vi "Jog Z_o.vi"(10 "array IN":dbl[](array[numeric]), 11 "Jog Cluster":T1={"Jog XY Cluster"={"object goes up"=FALSE, "object goes down"=FALSE, "object goes right"=FALSE, "object goes left"=FALSE, "SW2"=FALSE, "SW1"=FALSE, "YY (mm)"=0.1, "YN (mm) "=0.01, "NY (mm) "=0.005, "NN (mm) "=0.001}, "Jog Z Cluster "={"Z go down 0.1 mm"=FALSE, "Z go up 0.1 mm"=FALSE, "Z go down 0.05 mm"=FALSE, "Z go up 0.05 mm"=FALSE, "Z go down 0.01 mm"=FALSE, "Z go up 0.01 mm"=FALSE, "Z go down"=FALSE, "Z go up"=FALSE, "step (mm)"=0.001}}) -> (2 "array OUT":dbl[](array[numeric]), 3 "Jog Cluster 2":T1={"Jog XY Cluster"={"object goes up"=FALSE, "object goes down"=FALSE, "object goes right"=FALSE, "object goes left"=FALSE, "SW2"=FALSE, "SW1"=FALSE, "YY (mm)"=0.1, "YN (mm) "=0.01, "NY (mm) "=0.005, "NN (mm) "=0.001}, "Jog Z Cluster "={"Z go down 0.1 mm"=FALSE, "Z go up 0.1 mm"=FALSE, "Z go down 0.05 mm"=FALSE, "Z go up 0.05 mm"=FALSE, "Z go down 0.01 mm"=FALSE, "Z go up 0.01 mm"=FALSE, "Z go down"=FALSE, "Z go up"=FALSE, "step (mm)"=0.001}})   [LabVIEW 2016]
panel:
  out "output array":dbl[](array[numeric])
  out "element":dbl
  out "index of element":i32
  out "appended array":bool[](array[boolean])
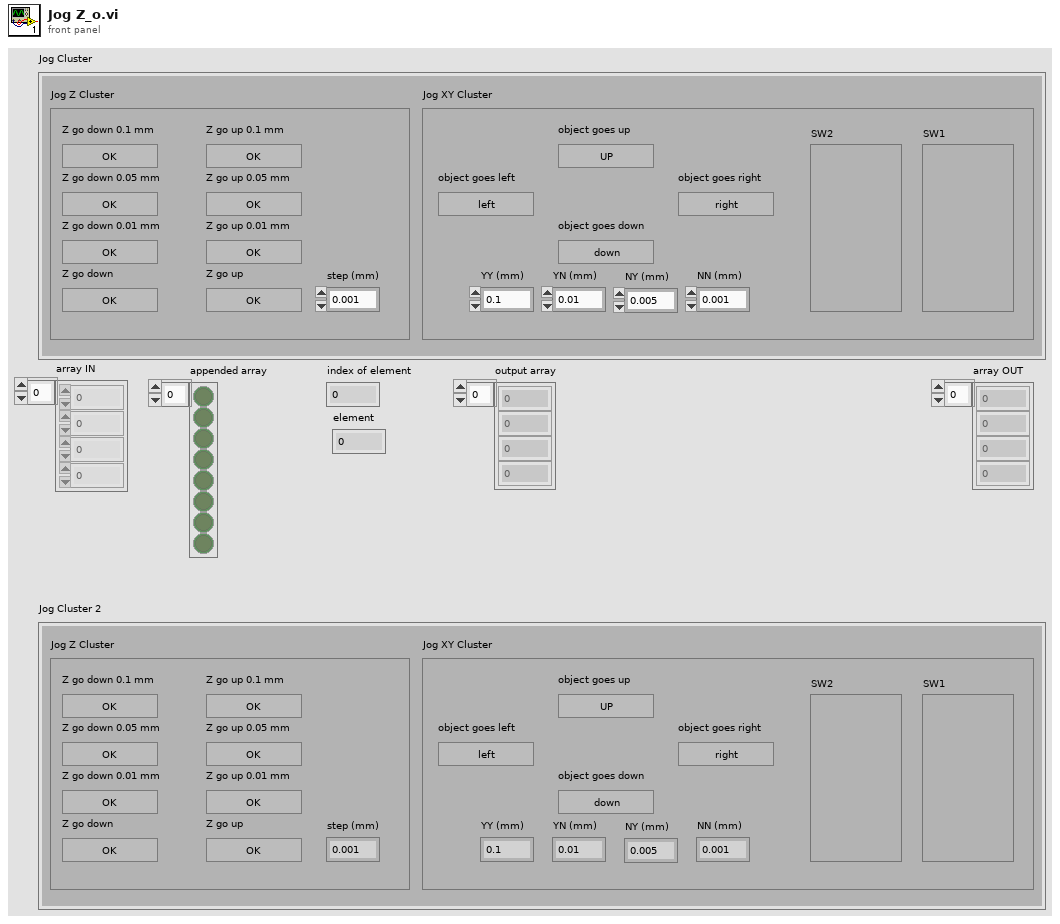
[diagram p1: front panel]
types:
  T1 = cluster{"Jog XY Cluster":cluster{"object goes up":bool, "object goes down":bool, "object goes right":bool, "object goes left":bool, "SW2":bool, "SW1":bool, "YY (mm)":dbl, "YN (mm) ":dbl, "NY (mm) ":dbl, "NN (mm) ":dbl}, "Jog Z Cluster ":cluster{"Z go down 0.1 mm":bool, "Z go up 0.1 mm":bool, "Z go down 0.05 mm":bool, "Z go up 0.05 mm":bool, "Z go down 0.01 mm":bool, "Z go up 0.01 mm":bool, "Z go down":bool, "Z go up":bool, "step (mm)":dbl}}
  T2 = cluster{"Z go down 0.1 mm":bool, "Z go up 0.1 mm":bool, "Z go down 0.05 mm":bool, "Z go up 0.05 mm":bool, "Z go down 0.01 mm":bool, "Z go up 0.01 mm":bool, "Z go down":bool, "Z go up":bool, "step (mm)":dbl}
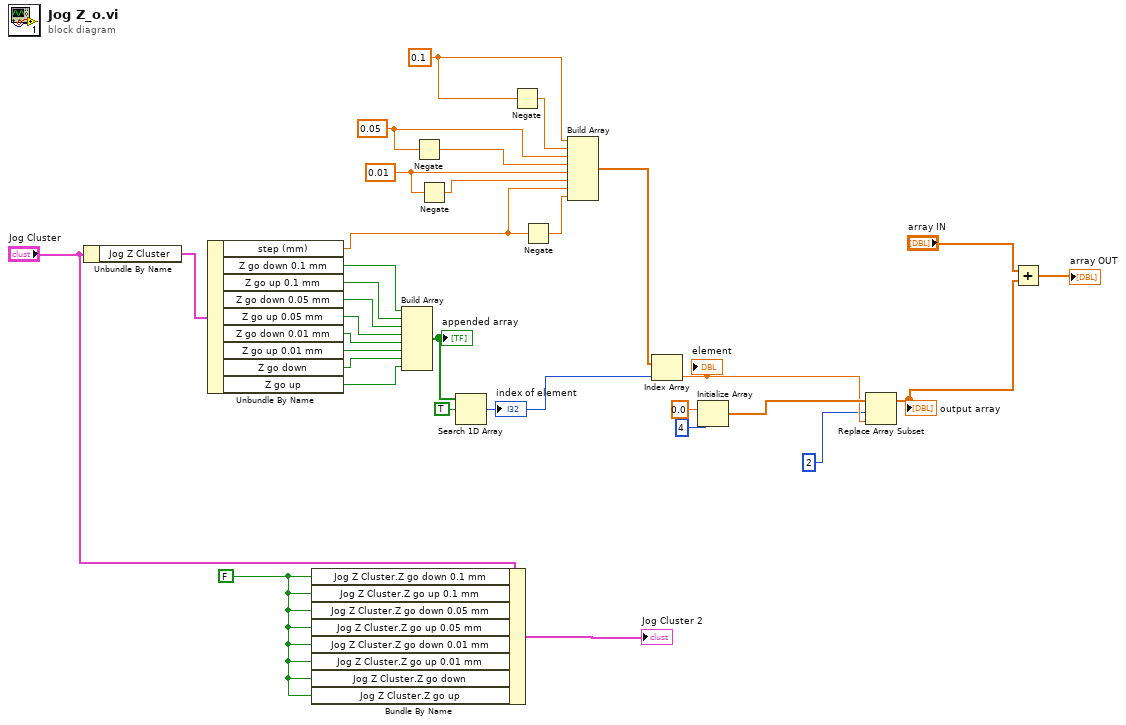
[diagram p0: block diagram]
diagram:
  w4 = FALSE ("Jog XY Cluster.object goes up")
  w8 = 0.01
  w6 = 0.05
  w12 = 0.1
  n1 = Unbundle By Name("Jog Cluster") -> ("Jog Z Cluster"=w2:T2)
  n2 = Unbundle By Name(w2) -> ("step (mm)"=w9:dbl, "Z go down 0.1 mm"=w21:bool, "Z go up 0.1 mm"=w20:bool, "Z go down 0.05 mm"=w19:bool, "Z go up 0.05 mm"=w18:bool, "Z go down 0.01 mm"=w17:bool, "Z go up 0.01 mm"=w16:bool, "Z go down"=w15:bool, "Z go up"=w14:bool)
  n3 = Bundle By Name(cluster="Jog Cluster", "Jog Z Cluster.Z go down 0.1 mm"=w4, "Jog Z Cluster.Z go up 0.1 mm"=w4, "Jog Z Cluster.Z go down 0.05 mm"=w4, "Jog Z Cluster.Z go up 0.05 mm"=w4, "Jog Z Cluster.Z go down 0.01 mm"=w4, "Jog Z Cluster.Z go up 0.01 mm"=w4, "Jog Z Cluster.Z go down"=w4, "Jog Z Cluster.Z go up"=w4) -> (→"Jog Cluster 2":T1)
  n4 = Build Array(w21, w20, w19, w18, w17, w16, w15, w14) -> (w26:bool[])
  "appended array" <- w26
  n5 = Negate(x=w6) -> (-x=w7:dbl)
  n6 = Negate(x=w8) -> (-x=w10:dbl)
  n7 = Search 1D Array(1D array=w26, element=TRUE) -> (index of element=w25:i32)  [unwired: 1 in]
  "index of element" <- w25
  n8 = Negate(x=w12) -> (-x=w13:dbl)
  n9 = Negate(x=w9) -> (-x=w11:dbl)
  n10 = Build Array(w12, w13, w6, w7, w8, w10, w9, w11) -> (w24:dbl[])
  n11 = Index Array(array=w24, index=w25) -> (element=w23:dbl)
  "element" <- w23
  n12 = Initialize Array(0.0 ("element"), 4 ("dimension size")) -> (w27:dbl[])
  n13 = Replace Array Subset(array=w27, new element=w23, index=2) -> (w30:dbl[])
  "output array" <- w30
  n14 = Add(x="array IN", y=w30) -> (x+y=→"array OUT":dbl[])
